vi "LKIF_DataStorageGetStatus.vi"(8 "error in (no error)":errorcluster {"code" format="%x"}, 11 "OutNo (0: OUT1)":i32) -> (0 "error out":errorcluster {"code" format="%x"}, 2 "NumStorageData":i32, 3 "IsStorage":bool)   [LabVIEW 2024, in "Keyence LK-G3000.lvlib"]
uses:
  Keyence LK-G3000.lvlib
  Keyance Demo Code/Keyence LK-G3000/LkIF.dll
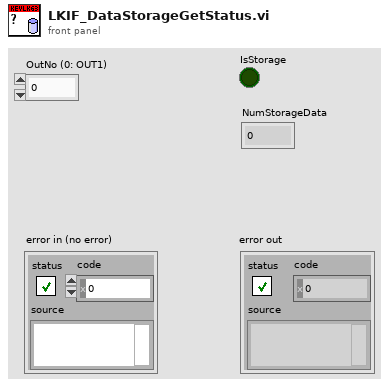
[diagram p1: front panel]
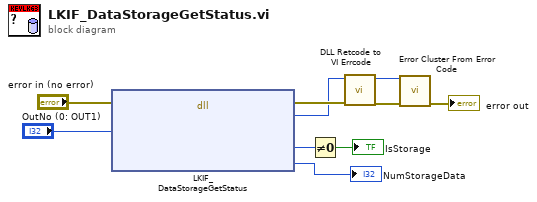
[diagram p0: block diagram]
diagram:
  n1 = dll-call lib="C:/Users/ff107/OneDrive/Documents/GitHub/PWC-OLS/Hardware Interface/Keyance Demo Code/Keyence LK-G3000/LkIF.dll" fn="LKIF_DataStorageGetStatus"(error in="error in (no error)", "OutNo"="OutNo (0: OUT1)") -> (error out=w6:errorcluster, "RC"=w5:i32, "IsStorage"=w4:i32, "NumStorageData"=→"NumStorageData":i32)  [unwired: 5 in, 1 out]
  n2 = Not Equal To 0?(x=w4) -> (x != 0?=→"IsStorage":bool)
  n3 = call "DLL Retcode to VI Errcode.vi"("error in (no error)"=w6, "DLL Retcode"=w5) -> ("error out"=w10:errorcluster, "VI Errcode"=w9:i32)  [unwired: 8 in]
  n4 = call <vilib>:"Error Cluster From Error Code.vi"("error in (no error)"=w10, "error code (0)"=w9) -> ("error out"=→"error out":errorcluster)  [unwired: 7 in]
